vi "Fit Line - 3D Test.vi"() -> ()   [LabVIEW 2023]
uses:
  Vec3d Class/Vec3d.lvclass
panel:
  out "centroid":cluster{"X":dbl, "Y":dbl, "Z":dbl}
  out "direction":cluster{"X":dbl, "Y":dbl, "Z":dbl}
  out "residual":dbl
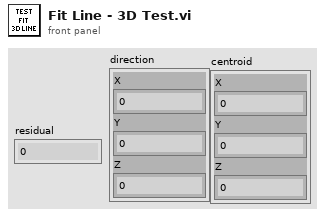
[diagram p1: front panel]
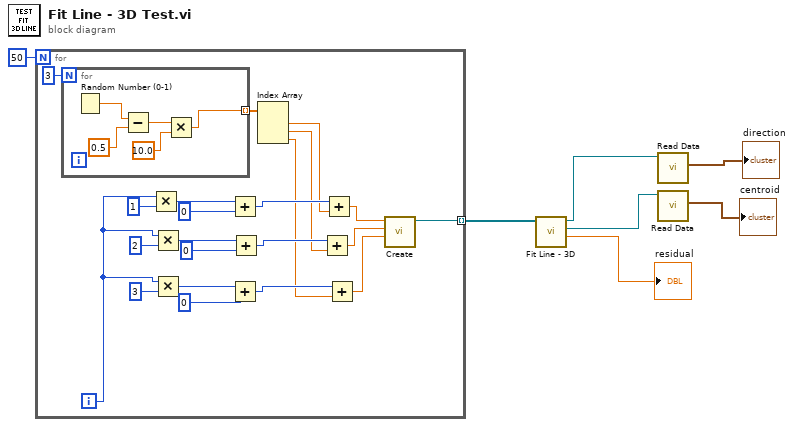
[diagram p0: block diagram]
diagram:
  n1 = for {
    N: 50 -> [_]
    tunnel: [w17] -> w6 mode=indexing
    i -> [w26]
    n2 = for {
      N: 3 -> [_]
      tunnel: [w31] -> w24 mode=indexing
      n3 = Random Number (0-1)() -> (number: 0 to 1=w34:dbl)
      n4 = Subtract(x=w34, y=0.5) -> (x-y=w32:dbl)
      n5 = Multiply(x=w32, y=10.0) -> (x*y=w31:dbl)
    }
    n6 = Multiply(x=w26, y=1) -> (x*y=w21:i32)
    n7 = Multiply(x=w26, y=2) -> (x*y=w22:i32)
    n8 = Multiply(x=w26, y=3) -> (x*y=w23:i32)
    n9 = Add(x=w21, y=0) -> (x+y=w16:i32)
    n10 = Add(x=w23, y=0) -> (x+y=w10:i32)
    n11 = Add(x=w22, y=0) -> (x+y=w13:i32)
    n12 = Index Array(array=w24) -> (element #1=w15:dbl, element #2=w12:dbl, element #3=w9:dbl)  [unwired: 3 in]
    n13 = Add(x=w13, y=w12) -> (x+y=w11:dbl)
    n14 = Add(x=w16, y=w15) -> (x+y=w14:dbl)
    n15 = Add(x=w10, y=w9) -> (x+y=w8:dbl)
    n16 = call "Create.vi"("Z"=w8, "Y"=w11, "X"=w14) -> ("Vec3d Class out"=w17:refnum<class "Vec3d.lvclass">)  [unwired: 7 in, 1 out]
  }
  n17 = call "Fit Line - 3D.vi"("Points"=w6) -> ("residual"=→"residual":dbl, "centroid"=w3:refnum<class "Vec3d.lvclass">, "direction"=w4:refnum<class "Vec3d.lvclass">)  [unwired: 7 in, 1 out]
  n18 = call-dynamic "Read Data.vi"("Vec3d Class in"=w4) -> ("Data"=→"direction":cluster{"X":dbl, "Y":dbl, "Z":dbl})  [unwired: 8 in, 2 out]
  n19 = call-dynamic "Read Data.vi"("Vec3d Class in"=w3) -> ("Data"=→"centroid":cluster{"X":dbl, "Y":dbl, "Z":dbl})  [unwired: 8 in, 2 out]
